vi "CMS_MODE - Type.vi"(8 "error in (no error)":errorcluster) -> (0 "error out":errorcluster, 3 "CMS_MODE_VALUE":i32)   [LabVIEW 2015]
doc: "<b>Buffer policy settings can be only unsafe in xiAPI LabVIEW library</b>\nUNSAFE : User gets pointer to internally allocated circle buffer and data may be overwritten by device.\nSAFE : Data from device will be copied to user allocated buffer or xiApi allocated memory."
uses:
  C:/GIT/Cameras3.x/Integrations/Labview/xiLib/xiLIB_32bit/xiLIB/xiCamLib/API/x86/xiApi.NET.dll
  xiLIB_32bit/xiLIB/xiCamLib/API/x86/xiApi.NET.dll
  CMS_MODE.ctl
panel:
  in  "CMS_MODE":T1
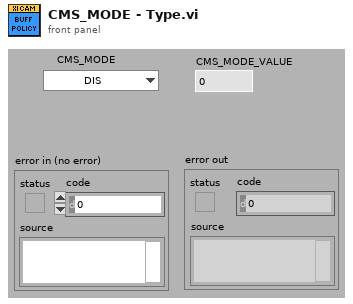
[diagram p1: front panel]
types:
  T1 = typedef "CMS_MODE.ctl" = enum16{"DIS", "EN", "EN_FAST"}
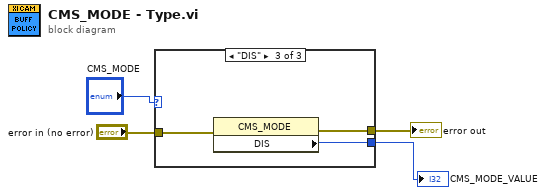
[diagram p0: block diagram]
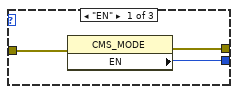
[diagram p2: hidden frame]
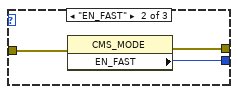
[diagram p3: hidden frame]
diagram:
  n1 = case shown="\"DIS\"" "CMS_MODE" {
    tunnel: "error in (no error)" -> [w7 w10 w13]
    tunnel: [w6 w9 w12] -> w3
    tunnel: [w5 w8 w11] -> w2
    frame "EN" {
      n2 = property class="CMS_MODE"(error in=w7) -> (error out=w6:errorcluster, "EN"=w5:i32)  [unwired: 1 in, 1 out]
    }
    frame "EN_FAST" {
      n3 = property class="CMS_MODE"(error in=w10) -> (error out=w9:errorcluster, "EN_FAST"=w8:i32)  [unwired: 1 in, 1 out]
    }
    frame "DIS" {
      n4 = property class="CMS_MODE"(error in=w13) -> (error out=w12:errorcluster, "DIS"=w11:i32)  [unwired: 1 in, 1 out]
    }
  }
  "error out" <- w3
  "CMS_MODE_VALUE" <- w2
